vi "numrowglobal.vi"() -> ()   [LabVIEW 2016]
panel:
  out "numrws":dbl format="%.2f"
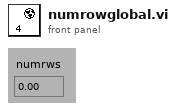
[diagram p1: front panel]
diagram:
